vi "MW setup_Ver1.vi"(11 "mw":T1={"mw_source"=enum."rigol", "MW Source IP Address"="169.254.101.2", "Remote Port"=18, "Frequency(MHz)"=1355.0, "Power(dBm)"=-27.0}) -> (2 "Currenct Power (dBm)":dbl=-30.0, 3 "Currenct Freqency (MHz)":dbl=1307.130243)   [LabVIEW 2020]
uses:
  mw.ctl
  Labview Library/Libraries/LaoJi/Logger/Send Error Message from VI.vi
panel:
  in  "read  source?":bool
  out "error out":errorcluster
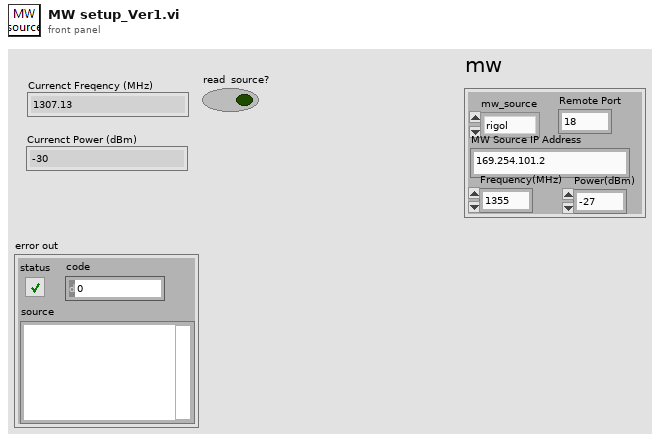
[diagram p1: front panel]
types:
  T1 = typedef "mw.ctl" = cluster{"mw_source":enum16{"rigol", "stanford", "apsin", "hittle"}, "MW Source IP Address":string, "Remote Port":u16, "Frequency(MHz)":dbl, "Power(dBm)":dbl}
  T2 = enum16{"Standard", "Buffered", "CRLF", "Immediate"}
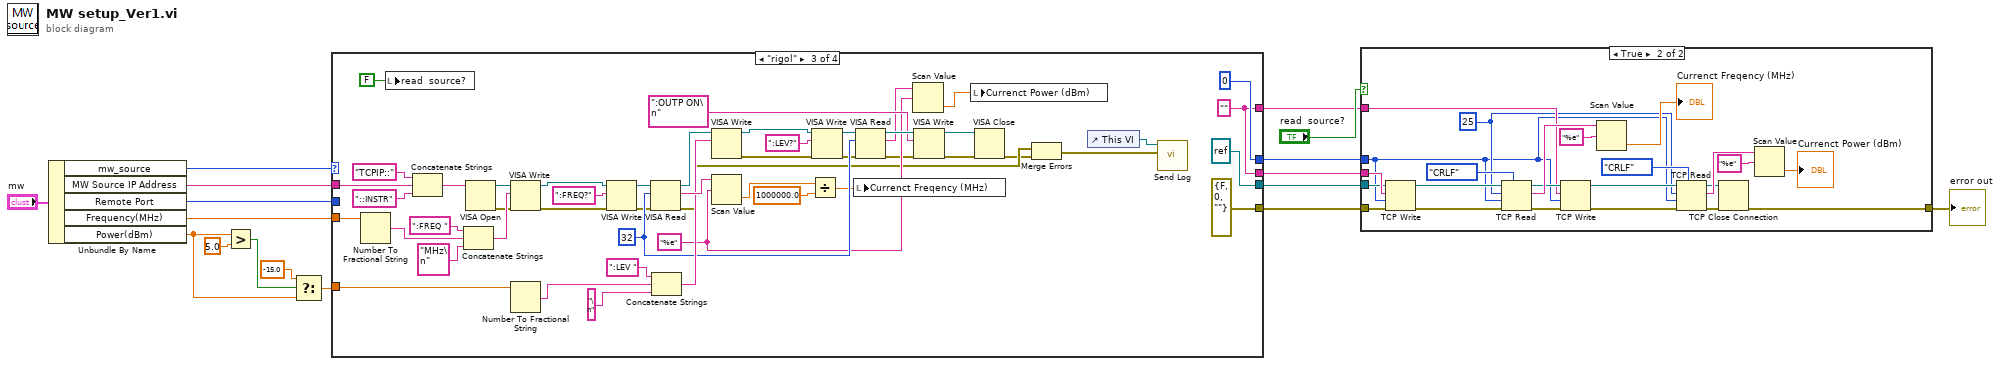
[diagram p0: block diagram]
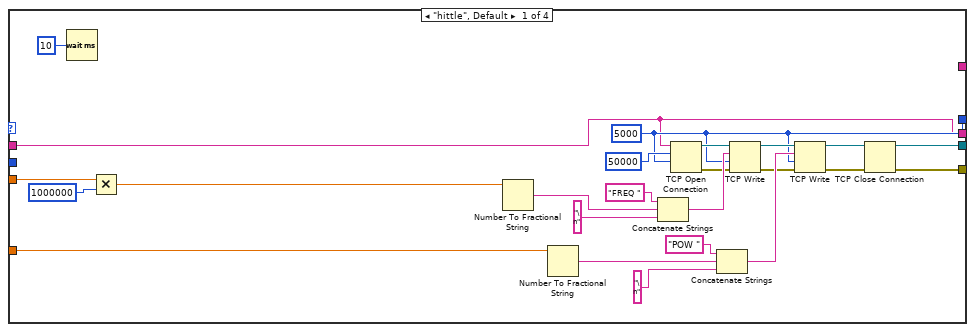
[diagram p2: hidden frame]
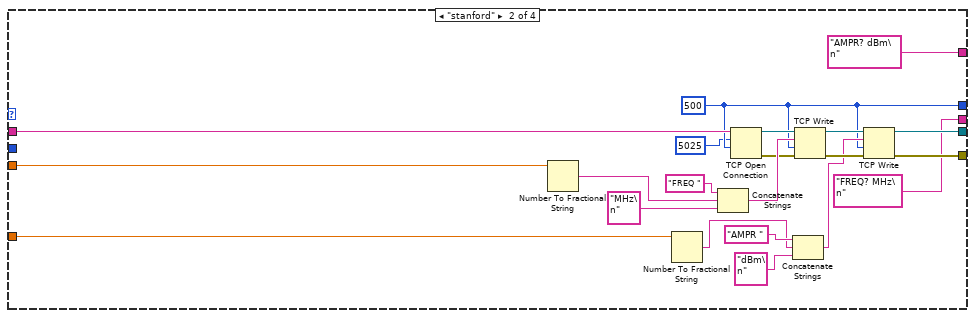
[diagram p3: hidden frame]
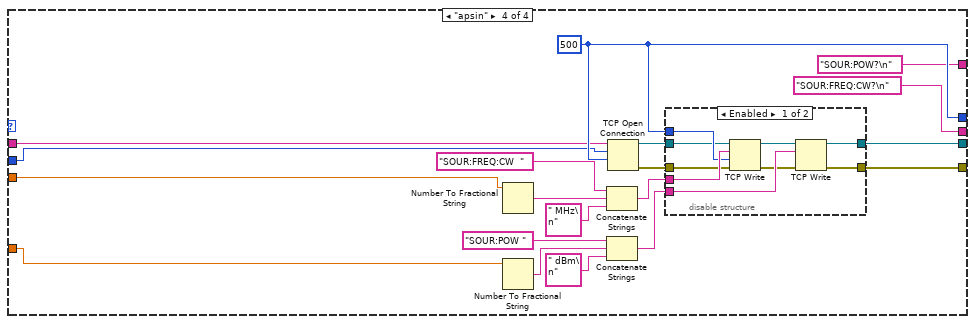
[diagram p4: hidden frame]
diagram:
  n1 = Unbundle By Name("mw") -> ("mw_source"=w9:enum16{"rigol", "stanford", "apsin", "hittle"}, "MW Source IP Address"=w12:string, "Remote Port"=w11:u16, "Frequency(MHz)"=w10:dbl, "Power(dBm)"=w2:dbl)
  n2 = Greater?(x=w2, y=5.0) -> (0:w4:bool)
  n3 = Select(t=-15.0, s=w4, f=w2) -> (s? t:f=w1:dbl)
  n4 = case shown="\"rigol\"" w9 {
    tunnel: [w18 "FREQ? MHz\n" w110 "SOUR:FREQ:CW?\n" ("数据输入")] -> w17
    tunnel: [w19 w48 errorcluster {"status"=FALSE, "code"=0, "source"=""} ("error out") w124] -> w16
    tunnel: [w20 w49 refnum<k5> refnum ("connection ID") w123] -> w15
    tunnel: [w21 w47 0 ("超时毫秒(60000)") w119] -> w14
    tunnel: w12 -> [w18 w59 w75 w116]
    tunnel: w11 -> [_ _ _ w115]
    tunnel: w10 -> [w22 w51 w105 w114]
    tunnel: w1 -> [w23 w52 w90 w113]
    tunnel: [_ "AMPR? dBm\n" w110 "SOUR:POW?\n" ("数据输入")] -> w8
    frame "hittle", Default {
      w21 = 5000 ("超时毫秒(60000)")
      n5 = Wait (ms)(milliseconds to wait=u32 10 ("等待时间（毫秒）")) -> ()  [unwired: 1 out]
      n6 = Multiply(x=w22, y=u32 1000000 ("等待时间（毫秒）")) -> (x*y=w28:dbl)
      n7 = Number To Fractional String(number=w28) -> (F-format string=w32:string)  [unwired: 3 in]
      n8 = Number To Fractional String(number=w23) -> (F-format string=w24:string)  [unwired: 3 in]
      n9 = Concatenate Strings("FREQ " ("数据输入"), w32, "\n" ("字符串")) -> (w39:string)
      n10 = TCP Open Connection(address=w18, remote port or service name=50000 ("超时毫秒(60000)"), timeout ms (60000)=w21) -> (connection ID=w31:refnum<k5>, error out=w30:errorcluster)  [unwired: 2 in]
      n11 = Concatenate Strings("POW " ("字符串"), w24, "\n" ("字符串")) -> (w34:string)
      n12 = TCP Write(connection ID=w31, data in=w39, error in (no error)=w30, 9:w21) -> (connection ID out=w35:refnum<k5>, error out=w33:errorcluster)  [unwired: 1 out]
      n13 = TCP Write(connection ID=w35, data in=w34, error in (no error)=w33, 9:w21) -> (connection ID out=w27:refnum<k5>, error out=w26:errorcluster)  [unwired: 1 out]
      n14 = TCP Close Connection(connection ID=w27, error in (no error)=w26) -> (connection ID out=w20:refnum<k5>, error out=w19:errorcluster)  [unwired: 1 in]
    }
    frame "stanford" {
      w47 = 500
      n15 = Number To Fractional String(number=w51) -> (F-format string=w61:string)  [unwired: 3 in]
      n16 = Number To Fractional String(number=w52) -> (F-format string=w53:string)  [unwired: 3 in]
      n17 = Concatenate Strings("FREQ ", w61, "MHz\n") -> (w57:string)
      n18 = TCP Open Connection(address=w59, remote port or service name=u16 5025, timeout ms (60000)=w47) -> (connection ID=w58:refnum<k5>, error out=w44:errorcluster)  [unwired: 2 in]
      n19 = Concatenate Strings("AMPR ", w53, "dBm\n" ("string")) -> (w50:string)
      n20 = TCP Write(connection ID=w58, data in=w57, error in (no error)=w44, 9:w47) -> (connection ID out=w56:refnum<k5>, error out=w55:errorcluster)  [unwired: 1 out]
      n21 = TCP Write(connection ID=w56, data in=w50, error in (no error)=w55, 9:w47) -> (connection ID out=w49:refnum<k5>, error out=w48:errorcluster)  [unwired: 1 out]
    }
    frame "rigol" {
      w84 = u32 32 ("byte count")
      w83 = "%e" ("格式字符串")
      w110 = "" ("数据输入")
      n22 = Number To Fractional String(number=w105) -> (F-format string=w102:string)  [unwired: 3 in]
      n23 = local write "read  source?"(FALSE ("read  source?")) -> ()
      n24 = Concatenate Strings("TCPIP::" ("string"), w75, "::INSTR" ("string")) -> (w74:string)
      n25 = Concatenate Strings(":FREQ " ("string"), w102, "MHz\n" ("string")) -> (w101:string)
      n26 = VISA Open(VISA resource name=w74) -> (VISA resource name=w106:refnum<visa-resource-name>, error out=w73:errorcluster)  [unwired: 4 in]
      n27 = VISA Write(VISA resource name=w106, write buffer=w101, error in (no error)=w73) -> (VISA resource name out=w99:refnum<visa-resource-name>, error out=w72:errorcluster)  [unwired: 1 out]
      n28 = Number To Fractional String(number=w90) -> (F-format string=w89:string)  [unwired: 3 in]
      n29 = VISA Write(VISA resource name=w99, write buffer=":FREQ?", error in (no error)=w72) -> (VISA resource name out=w98:refnum<visa-resource-name>, error out=w71:errorcluster)  [unwired: 1 out]
      n30 = VISA Read(VISA resource name=w98, byte count=w84, error in (no error)=w71) -> (VISA resource name out=w96:refnum<visa-resource-name>, read buffer=w97:string, error out=w66:errorcluster)  [unwired: 1 out]
      n31 = Concatenate Strings(":LEV " ("string"), w89, "\n" ("string")) -> (w86:string)
      n32 = VISA Write(VISA resource name=w96, write buffer=w86) -> (VISA resource name out=w95:refnum<visa-resource-name>, error out=w70:errorcluster)  [unwired: 1 in, 1 out]
      n33 = Scan Value(string=w97, format string=w83) -> (value=w79:dbl)  [unwired: 1 in, 1 out]
      n34 = Divide(x=w79, y=1000000.0) -> (x/y=w78:dbl)
      n35 = VISA Write(VISA resource name=w95, write buffer=":LEV?", error in (no error)=w70) -> (VISA resource name out=w94:refnum<visa-resource-name>, error out=w69:errorcluster)  [unwired: 1 out]
      n36 = local write "Currenct Freqency (MHz)"(w78) -> ()
      n37 = VISA Read(VISA resource name=w94, byte count=w84, error in (no error)=w69) -> (VISA resource name out=w93:refnum<visa-resource-name>, read buffer=w82:string, error out=w68:errorcluster)  [unwired: 1 out]
      n38 = Scan Value(string=w82, format string=w83) -> (value=w81:dbl)  [unwired: 1 in, 1 out]
      n39 = VISA Write(VISA resource name=w93, write buffer=":OUTP ON\n", error in (no error)=w68) -> (VISA resource name out=w92:refnum<visa-resource-name>, error out=w67:errorcluster)  [unwired: 1 out]
      n40 = local write "Currenct Power (dBm)"(w81) -> ()
      n41 = VISA Close(VISA resource name=w92, error in (no error)=w67) -> (error out=w65:errorcluster)
      n42 = Merge Errors(w66, w65) -> (w64:errorcluster)
      n43 = control-ref of="This VI"() -> (w63:refnum<vi>)
      n44 = call-poly "Send Log.vi"("Message"=w64, "VI Refnum"=w63) -> ()  [unwired: 8 in, 2 out]
    }
    frame "apsin" {
      w119 = 500 ("超时毫秒(60000)")
      n45 = Number To Fractional String(number=w114) -> (F-format string=w121:string)  [unwired: 3 in]
      n46 = Number To Fractional String(number=w113) -> (F-format string=w120:string)  [unwired: 3 in]
      n47 = Concatenate Strings("SOUR:FREQ:CW  " ("数据输入"), w121, " MHz\n" ("字符串")) -> (w127:string)
      n48 = Concatenate Strings("SOUR:POW " ("字符串"), w120, " dBm\n" ("字符串")) -> (w122:string)
      n49 = TCP Open Connection(address=w116, remote port or service name=w115, timeout ms (60000)=w119) -> (connection ID=w118:refnum<k5>, error out=w117:errorcluster)  [unwired: 2 in]
      n50 = disable-structure shown="Enabled" {
        disable-tunnel: w127 -> [w139 _]
        disable-tunnel: [w138 w140] -> w124
        disable-tunnel: [w136 w141] -> w123
        disable-tunnel: w122 -> [w135 _]
        disable-tunnel: w119 -> [w133 _]
        disable-tunnel: w118 -> [w132 w141]
        disable-tunnel: w117 -> [w131 w140]
        frame Enabled {
          n51 = TCP Write(connection ID=w132, data in=w139, error in (no error)=w131, 9:w133) -> (connection ID out=w137:refnum<k5>, error out=w134:errorcluster)  [unwired: 1 out]
          n52 = TCP Write(connection ID=w137, data in=w135, error in (no error)=w134) -> (connection ID out=w136:refnum<k5>, error out=w138:errorcluster)  [unwired: 1 in, 1 out]
        }
        frame Disabled {
        }
      }
    }
  }
  n53 = case shown="True" "read  source?" {
    tunnel: w17 -> [_ w165]
    tunnel: w16 -> [w142 w160]
    tunnel: w15 -> [_ w159]
    tunnel: w14 -> [_ w146]
    tunnel: w8 -> [_ w148]
    tunnel: [w142 w143] -> w6
    frame False {
    }
    frame True {
      w147 = 25 ("读取的字节")
      n54 = TCP Write(connection ID=w159, data in=w165, error in (no error)=w160, 9:w146) -> (connection ID out=w163:refnum<k5>, error out=w164:errorcluster)  [unwired: 1 out]
      n55 = TCP Read(connection ID=w163, bytes to read=w147, error in (no error)=w164, 7:T2."CRLF" ("mode (standard)"), 9:w146) -> (connection ID out=w153:refnum<k5>, data out=w162:string, error out=w152:errorcluster)
      n56 = TCP Write(connection ID=w153, data in=w148, error in (no error)=w152, 9:w146) -> (connection ID out=w155:refnum<k5>, error out=w154:errorcluster)  [unwired: 1 out]
      n57 = Scan Value(string=w162, format string="%e" ("格式字符串")) -> (value=→"Currenct Freqency (MHz)":dbl)  [unwired: 1 in, 1 out]
      n58 = TCP Read(connection ID=w155, bytes to read=w147, error in (no error)=w154, 7:T2."CRLF" ("mode (standard)"), 9:w146) -> (connection ID out=w144:refnum<k5>, data out=w149:string, error out=w145:errorcluster)
      n59 = TCP Close Connection(connection ID=w144, error in (no error)=w145) -> (error out=w143:errorcluster)  [unwired: 1 in, 1 out]
      n60 = Scan Value(string=w149, format string="%e" ("格式字符串")) -> (value=→"Currenct Power (dBm)":dbl)  [unwired: 1 in, 1 out]
    }
  }
  "error out" <- w6
